vi "Trap1-06-06-2017.vi"() -> (4 "U_MW":fxp<+/-,26,5> format="%.23g")   [LabVIEW 2010]
uses:
  <vilib>/eio/EIONode/EIONode.xnode
  <vilib>/rvi/eio/nirviEIOImplementation/nirviEIOImplementation.xnode
  <vilib>/rvi/eio/common/nirviEmuClasses.ctl
  <vilib>/rvi/FXPMathLib/FxpAdd/XNode/nifxpmath_Add.xnode
  <vilib>/rvi/FXPMathLib/FxpAdd/subVIs/nifxpmath_Add_SimConfig.ctl
  <vilib>/fxp/LVFixedPointQuantizationPolicyTypeDef.ctl
  <vilib>/fxp/LVFixedPointOverflowPolicyTypeDef.ctl
  <vilib>/rvi/FXPMathLib/FxpDiv/XNode/nifxpmath_Div.xnode
  <vilib>/rvi/FXPMathLib/FxpDiv/subVIs/nifxpmath_Div_SimConfig.ctl
  <vilib>/rvi/FXPMathLib/FxpSub/XNode/nifxpmath_Sub.xnode
  <vilib>/rvi/FXPMathLib/FxpSub/subVIs/nifxpmath_Sub_SimConfig.ctl
  <vilib>/rvi/FXPMathLib/FxpMul/XNode/nifxpmath_Multiplier.xnode
  <vilib>/rvi/FXPMathLib/FxpMul/subVIs/nifxpmath_Mul_SimConfig.ctl
  <vilib>/rvi/eio/common/nirviEmuTemplateMethod_noerrors.vi
  <vilib>/rvi/FXPMathLib/FxpAdd/simVIs/DllFxpAddTemp_sub.vi
  <vilib>/rvi/FXPMathLib/FxpDiv/simVIs/DllFxpDivTemp_sub.vi
  <vilib>/rvi/FXPMathLib/FxpSub/simVIs/DllFxpSubTemp_sub.vi
  <vilib>/rvi/FXPMathLib/FxpMul/simVIs/DllFxpMulTemp_sub.vi
panel:
  in  "Warten(uSec)":u16=5000
  out "PTStirling":fxp<+/-,26,5> format="%.23g"
  in  "Stirling":bool
  out "PreCol1_MW":fxp<+/-,26,5> format="%.23g"
  in  "d0":fxp<+/-,18,18> format="%.16g"
  in  "d1":fxp<+/-,21,21> format="%.16g"
  in  "U_SP":fxp<+/-,26,5> format="%.23g"
  in  "heizen":bool
  in  "stop":bool
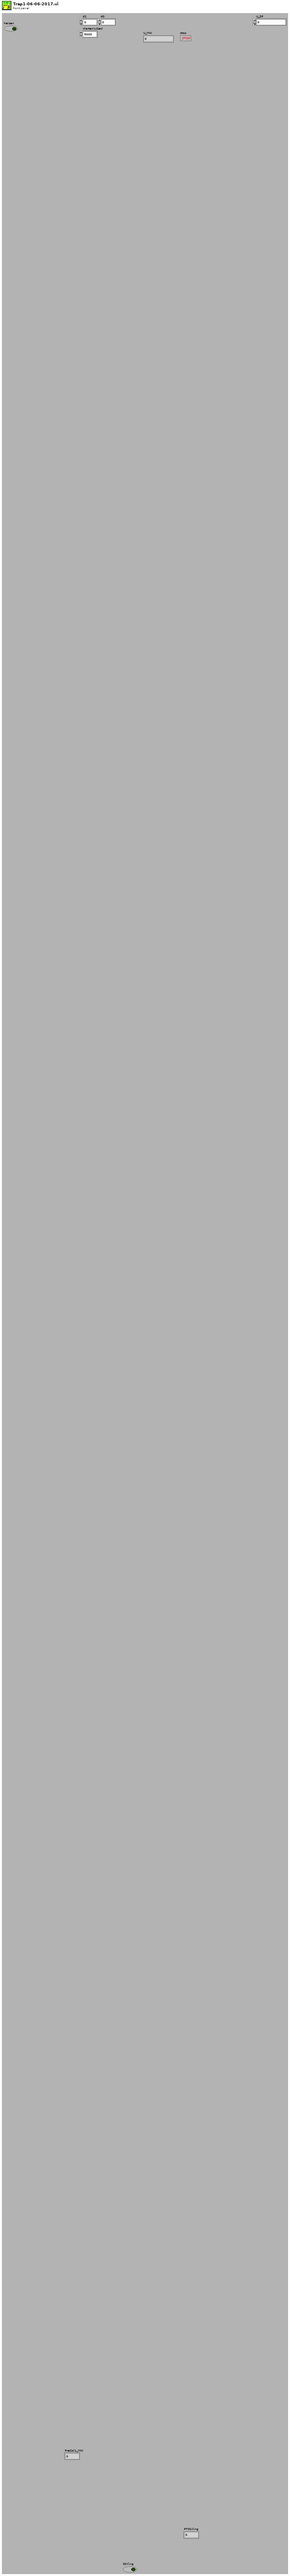
[diagram p1: front panel]
types:
  T1 = typedef "nirviEmuClasses.ctl" = enum16{"IO Read", "IO Write", "Method", "Property Read", "Property Write"}
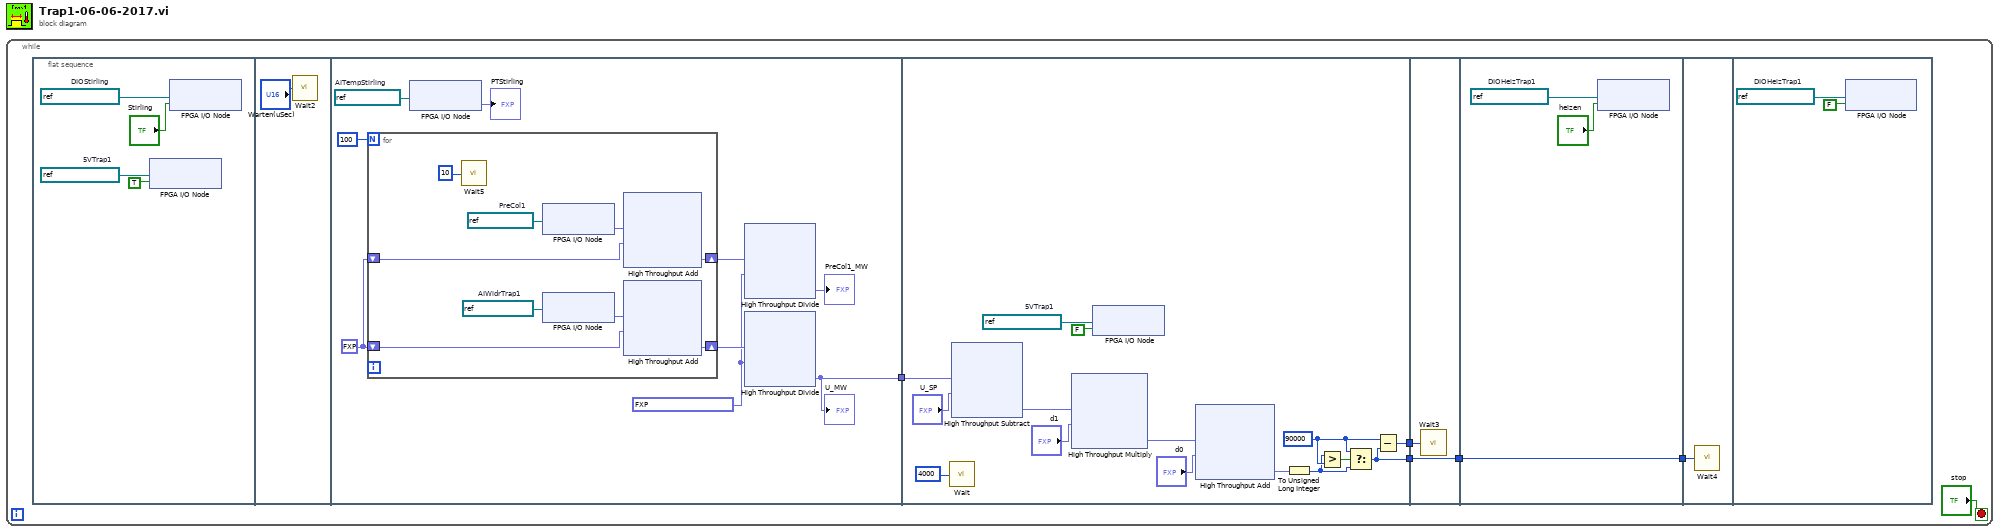
[diagram p0: block diagram]
diagram:
  n1 = while {
    stop <- "stop" stop-if-true
    n2 = flat-sequence {
      tunnel: [w40] -> w5
      tunnel: w5 -> [w233]
      tunnel: [w223] -> w2
      tunnel: [w227] -> w1
      tunnel: [w337] -> w3
      tunnel: w2 -> [w337]
      tunnel: w1 -> [w336]
      tunnel: [w338] -> w4
      tunnel: w3 -> [w338]
      tunnel: w4 -> [w352]
      frame #0 {
        w7 = refnum<k21> "Mod6/DIO12"  # DIOStirling
        w10 = refnum<k21> "Mod6/DIO21"  # 5VTrap1
        n3 = xnode "FPGA I/O Node"("I/O Item"=TRUE, "FPGA I/O In"=w10) -> ()  [unwired: 1 out]
        n4 = xnode "FPGA I/O Node"("I/O Item"="Stirling", "FPGA I/O In"=w7) -> ()  [unwired: 1 out]
      }
      frame #1 {
        n5 = call "Wait2"("Count(uSec)"="Warten(uSec)") -> ()  [unwired: 1 out]
      }
      frame #2 {
        w34 = refnum<k21> "Mod1/AI2"  # AITempStirling
        w37 = fxp<+/-,8,8> 100.0 ("y")
        w39 = fxp<+/-,33,12> 0.0 ("x+y")
        n6 = for {
          N: 100 -> [_]
          shift-right: [w120] -> w42
          shift-left: w39 -> [w121]
          shift-right: [w116] -> w38
          shift-left: w39 -> [w117]
          w119 = refnum<k21> "Mod1/AI3"  # PreCol1
          w124 = refnum<k21> "Mod1/AI30"  # AIWidrTrap1
          n7 = call "Wait5"("Count(uSec)"=u8 10) -> ()  [unwired: 1 out]
          n8 = xnode "FPGA I/O Node"("FPGA I/O In"=w119) -> ("I/O Item"=w118:fxp<+/-,26,5>)  [unwired: 1 out]
          n9 = xnode "FPGA I/O Node"("FPGA I/O In"=w124) -> ("I/O Item"=w122:fxp<+/-,26,5>)  [unwired: 1 out]
          n10 = xnode "High Throughput Add"("x"=w118, "y"=w117) -> ("x+y"=w116:fxp<+/-,33,12>)
          n11 = xnode "High Throughput Add"("x"=w122, "y"=w121) -> ("x+y"=w120:fxp<+/-,33,12>)
        }
        n12 = xnode "FPGA I/O Node"("FPGA I/O In"=w34) -> ("I/O Item"=→"PTStirling":fxp<+/-,26,5>)  [unwired: 1 out]
        n13 = xnode "High Throughput Divide"("x"=w38, "y"=w37) -> ("x/y"=→"PreCol1_MW":fxp<+/-,26,5>)
        n14 = xnode "High Throughput Divide"("x"=w42, "y"=w37) -> ("x/y"=w40:fxp<+/-,26,5>)
        "U_MW" <- w40
      }
      frame #3 {
        w225 = u32 90000 ("x")
        w237 = refnum<k21> "Mod6/DIO21"  # 5VTrap1
        n15 = call "Wait"("Count(uSec)"=u16 4000) -> ()  [unwired: 1 out]
        n16 = xnode "High Throughput Subtract"("x"=w233, "y"="U_SP") -> ("x-y"=w232:fxp<+/-,26,5>)
        n17 = xnode "High Throughput Multiply"("x"=w232, "y"="d1") -> ("x*y"=w230:fxp<+/-,18,18>)
        n18 = xnode "FPGA I/O Node"("I/O Item"=FALSE, "FPGA I/O In"=w237) -> ()  [unwired: 1 out]
        n19 = xnode "High Throughput Add"("x"=w230, "y"="d0") -> ("x+y"=w228:fxp<+/-,18,18>)
        n20 = To Unsigned Long Integer(number=w228) -> (unsigned 32bit integer=w224:u32)
        n21 = Greater?(x=w224, y=w225) -> (0:w226:bool)
        n22 = Select(t=w225, s=w226, f=w224) -> (s? t:f=w223:u32)
        n23 = Subtract(x=w225, y=w223) -> (x-y=w227:u32)
      }
      frame #4 {
        n24 = call "Wait3"("Count(uSec)"=w336) -> ()  [unwired: 1 out]
      }
      frame #5 {
        w340 = refnum<k21> "Mod6/DIO19"  # DIOHeizTrap1
        n25 = xnode "FPGA I/O Node"("I/O Item"="heizen", "FPGA I/O In"=w340) -> ()  [unwired: 1 out]
      }
      frame #6 {
        n26 = call "Wait4"("Count(uSec)"=w352) -> ()  [unwired: 1 out]
      }
      frame #7 {
        w354 = refnum<k21> "Mod6/DIO19"  # DIOHeizTrap1
        n27 = xnode "FPGA I/O Node"("I/O Item"=FALSE, "FPGA I/O In"=w354) -> ()  [unwired: 1 out]
      }
    }
  }
